vi "Write Rate (Hz).vi"(8 "error in":errorcluster, 10 "Rate (Hz)":i32, 11 "Reset Blue Laser Rep Rate in":refnum<class "Reset Blue Laser Rep Rate.lvclass">) -> (0 "error out":errorcluster, 3 "Reset Blue Laser Rep Rate out":refnum<class "Reset Blue Laser Rep Rate.lvclass">)   [LabVIEW 2014, in "eCRDS Library.lvlib" / "Reset Blue Laser Rep Rate.lvclass"]
uses:
  Reset Blue Laser Rep Rate.lvclass
  Reset Blue Laser Rep Rate.lvclass/Reset Blue Laser Rep Rate.ctl
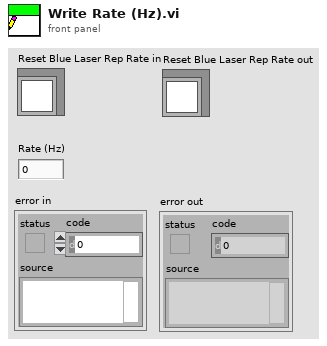
[diagram p1: front panel]
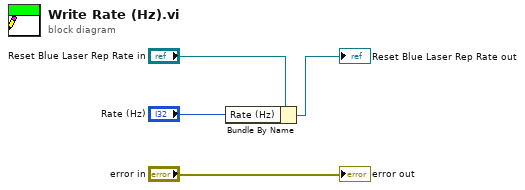
[diagram p0: block diagram]
diagram:
  n1 = Bundle By Name(cluster="Reset Blue Laser Rep Rate in", "Rate (Hz)"="Rate (Hz)") -> (→"Reset Blue Laser Rep Rate out":refnum<class "Reset Blue Laser Rep Rate.lvclass">)
  "error out" <- "error in"
